vi "nominal ingest tabular set timestamp custom.vi"(6 "default_day_of_year":i32, 7 "default_year":i32, 8 "error in (no error)":errorcluster, 9 "format":string, 10 "column":string, 11 "staging":i32) -> (0 "error out":errorcluster, 3 "function return":i32)   [LabVIEW 2020, in "client.lvlib"]
doc: "int32_t nominal_ingest_tabular_set_timestamp_custom(int32_t staging,\n const char *column,\n const char *format,\n int32_t default_year,\n int32_t default_day_of_year);"
uses:
  client.lvlib
  bin/nominalClient_64.dll
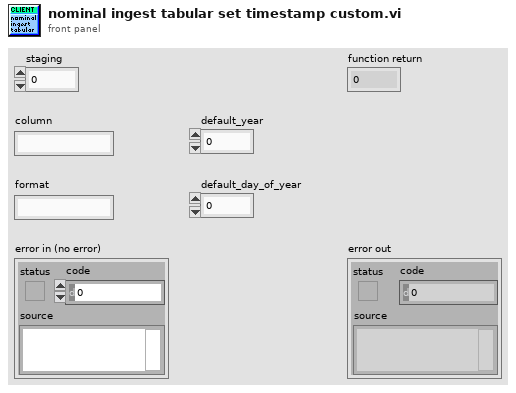
[diagram p1: front panel]
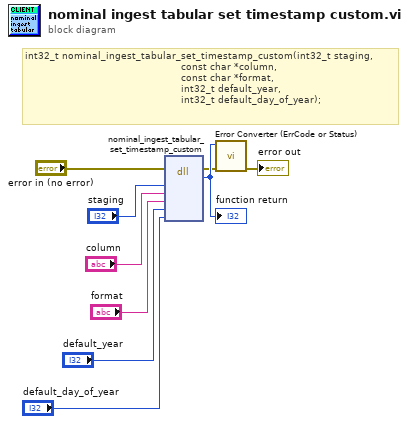
[diagram p0: block diagram]
diagram:
  # "int32_t nominal_ingest_tabular_set_timestamp_custom(int32_t staging,\n                                                    const char *column,\n                                                    const char *format,\n                                                    int32_t default_year,\n                                                    int32_t default_day_of_year);"
  n1 = dll-call lib="C:/code/labview-client-rs/lv_src/bin/nominalClient_*.*" fn="nominal_ingest_tabular_set_timestamp_custom"(error in="error in (no error)", "staging"="staging", "column"="column", "format"="format", "default_year"="default_year", "default_day_of_year"="default_day_of_year") -> (error out=w2:errorcluster, w9:i32)  [unwired: 7 in, 1 out]
  "function return" <- w9
  n2 = call "Error Converter (ErrCode or Status).vi"("error in (no error)"=w2, "error code"=w9) -> ("error out"=→"error out":errorcluster)  [unwired: 9 in]
